vi "armControl.vi"(8 "shooterAngleSetPoint":dbl format="%.2f", 9 "shooterAngleSensorOutput":dbl format="%.2f", 10 "lowerBound":dbl, 11 "upperBound":dbl) -> (0 "shooterAngleMotorOutput":dbl format="%.2f", 6 "shooterAnglePIDGains":T1={"proportional gain (Kc)"=1.0, "integral time (Ti, min)"=0.01, "derivative time (Td, min)"=0.0} {"derivative time (Td, min)" format="%.3f"; "integral time (Ti, min)" format="%.3f"; "proportional gain (Kc)" format="%.3f"})   [LabVIEW 2012]
uses:
  <vilib>/addons/control/pid/pid.llb/PID (DBL).vi
  <vilib>/addons/control/pid/NI_PID_pid.lvlib
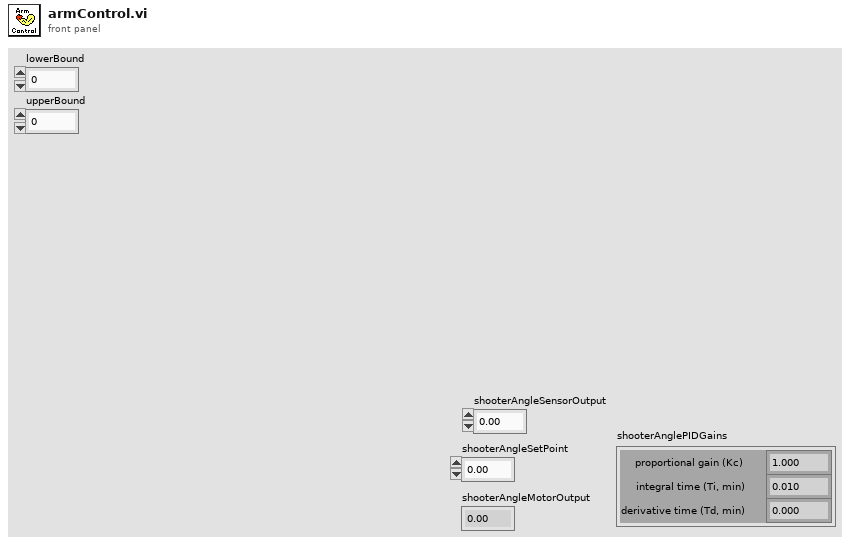
[diagram p1: front panel]
types:
  T1 = cluster{"proportional gain (Kc)":dbl, "integral time (Ti, min)":dbl, "derivative time (Td, min)":dbl}
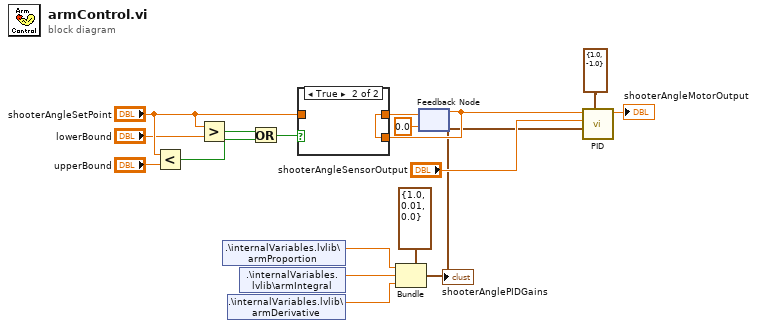
[diagram p0: block diagram]
diagram:
  n1 = Less?(x="shooterAngleSetPoint", y="upperBound") -> (x < y?=w16:bool)
  n2 = Greater?(x="shooterAngleSetPoint", y="lowerBound") -> (0:w17:bool)
  n3 = shared-variable ".\\internalVariables.lvlib\\armProportion"() -> (w4:dbl)  [unwired: 1 in, 1 out]
  n4 = shared-variable ".\\internalVariables.lvlib\\armDerivative"() -> (w3:dbl)  [unwired: 1 in, 1 out]
  n5 = shared-variable ".\\internalVariables.lvlib\\armIntegral"() -> (w2:dbl)  [unwired: 1 in, 1 out]
  n6 = Or(x=w17, y=w16) -> (x .or. y?=w15:bool)
  n7 = Bundle(cluster=T1 {"proportional gain (Kc)"=1.0, "integral time (Ti, min)"=0.01, "derivative time (Td, min)"=0.0} ("shooterAnglePIDGains"), "proportional gain (Kc)"=w4, "integral time (Ti, min)"=w2, "derivative time (Td, min)"=w3) -> (w1:T1)
  "shooterAnglePIDGains" <- w1
  n8 = feedback #1(0.0 ("shooterAngleSetPoint 2")) -> (w12:dbl)
  n9 = case shown="True" w15 {
    tunnel: "shooterAngleSetPoint" -> [w18 _]
    tunnel: [w18 w19] -> w13
    tunnel: w12 -> [_ w19]
    frame False {
    }
    frame True {
    }
  }
  n10 = feedback-in #1(w13) -> ()
  n11 = call-poly <vilib>:"PID.vi"("output range"=cluster{"output high":dbl, "output low":dbl} {"output high"=1.0, "output low"=-1.0}, "PID gains"=w1, "process variable"="shooterAngleSensorOutput", "setpoint"=w12) -> ("output"=→"shooterAngleMotorOutput":dbl)  [unwired: 6 in, 1 out]
